vi "Write rec0MQ.vi"(8 "error in (no error)":errorcluster, 10 "rec0MQ":bool, 11 "Messenger in":refnum<class "Messenger.lvclass">) -> (0 "error out":errorcluster, 3 "Messenger out":refnum<class "Messenger.lvclass">)   [LabVIEW 2018, in "Messenger.lvclass"]
uses:
  Messenger.lvclass
  Messenger.lvclass/Messenger.ctl
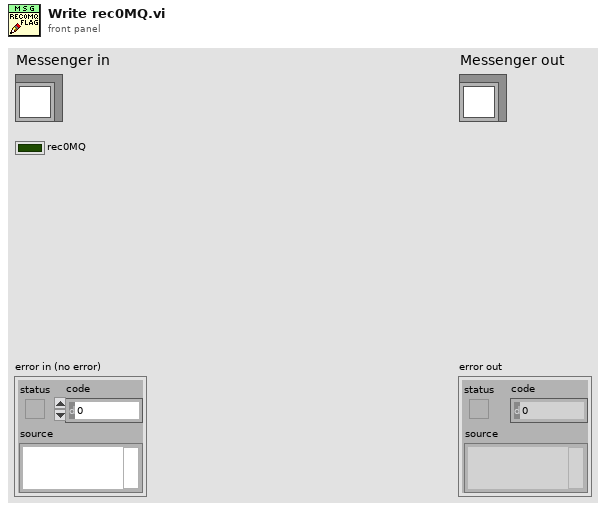
[diagram p1: front panel]
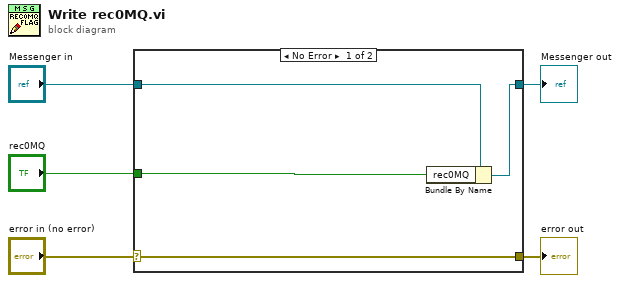
[diagram p0: block diagram]
diagram:
  n1 = case shown="No Error" "error in (no error)" {
    selector: "error in (no error)" -> [w9 w10]
    tunnel: [w9 w10] -> w4
    tunnel: [w7 w11] -> w2
    tunnel: "Messenger in" -> [w8 w11]
    tunnel: "rec0MQ" -> [w6 _]
    frame No Error {
      n2 = Bundle By Name(cluster=w8, "rec0MQ"=w6) -> (w7:refnum<class "Messenger.lvclass">)
    }
    frame Error {
    }
  }
  "error out" <- w4
  "Messenger out" <- w2
